vi "JSON - Replace Equals Character with Colon.vi"(8 "error in":errorcluster, 11 "Input JSON String":string) -> (0 "error out":errorcluster, 3 "Output JSON String":string)   [LabVIEW 2021]
doc: "Processes the JSON text by replacing and '=' characters with ':'"
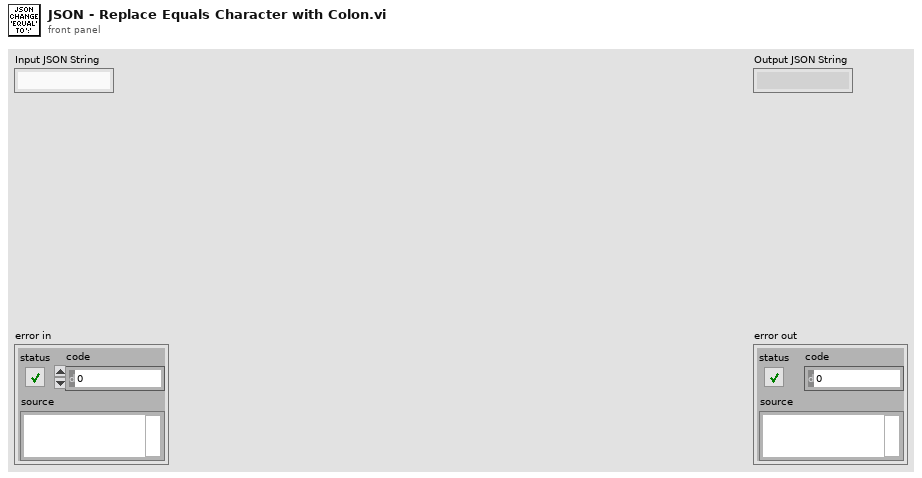
[diagram p1: front panel]
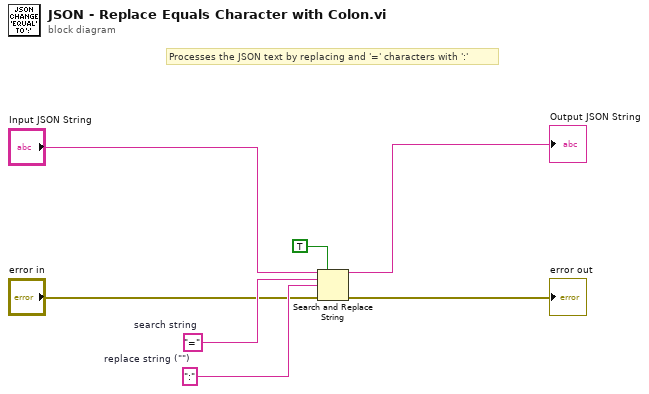
[diagram p0: block diagram]
diagram:
  w5 = ":"  # replace string ("")
  w6 = "="  # search string
  # "Processes the JSON text by replacing and '=' characters with ':'"
  n1 = Search and Replace String(replace all?=TRUE ("replace all? (F)"), input string="Input JSON String", search string=w6, replace string=w5, error in="error in") -> (result string=→"Output JSON String":string, error out=→"error out":errorcluster)  [unwired: 3 in, 2 out]
